vi "Position.vi"(8 "error in (no error)":errorcluster, 11 "Number in":refnum<class "Number.lvclass">) -> (0 "error out":errorcluster, 2 "Position":T1[](array[typedef]), 3 "Number out":refnum<class "Number.lvclass">)   [LabVIEW 2020, in "Number.lvclass"]
uses:
  Number.lvclass
  Coordinate.ctl
  Number.lvclass/Number.ctl
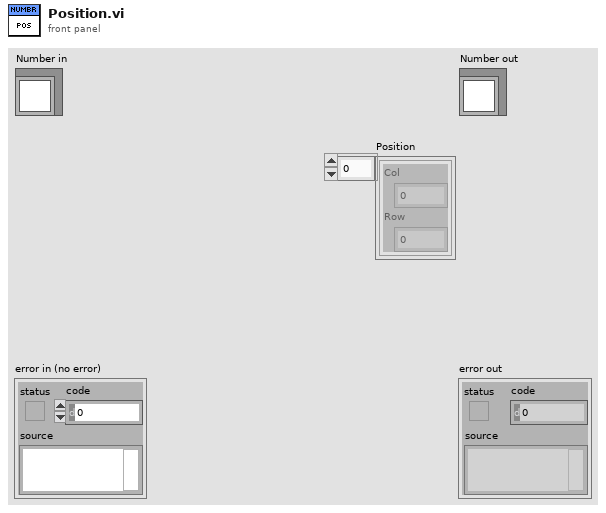
[diagram p1: front panel]
types:
  T1 = typedef "Number.lvclass/Coordinate.ctl" = cluster{"Col":i32, "Row":i32}
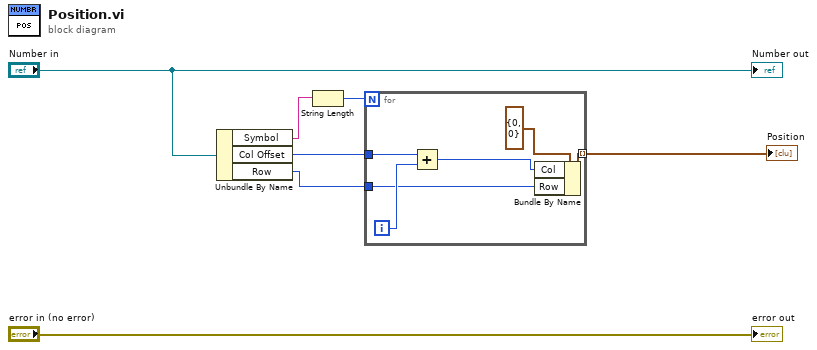
[diagram p0: block diagram]
diagram:
  n1 = Unbundle By Name("Number in") -> ("Symbol"=w4:string, "Col Offset"=w3:i32, "Row"=w1:i32)
  n2 = String Length(string=w4) -> (length=w5:i32)
  n3 = for {
    N: w5 -> [_]
    tunnel: w3 -> [w13]
    tunnel: [w10] -> w2 mode=indexing
    tunnel: w1 -> [w8]
    i -> [w12]
    n4 = Add(x=w13, y=w12) -> (x+y=w9:i32)
    n5 = Bundle By Name(cluster=T1 {"Col"=0, "Row"=0} ("Position"), "Col"=w9, "Row"=w8) -> (w10:T1)
  }
  "Position" <- w2
  "error out" <- "error in (no error)"
  "Number out" <- "Number in"
